vi "Memory.Pointer.Copy All.Unsafe.vi"(8 "error in (no error)":errorcluster, 10 "dst pointer in":refnum<class "Memory.Pointer.lvclass">, 11 "src pointer in":refnum<class "Memory.Pointer.lvclass">) -> (0 "error out":errorcluster, 2 "dst pointer out":refnum<class "Memory.Pointer.lvclass">, 3 "src pointer out":refnum<class "Memory.Pointer.lvclass">)   [LabVIEW 2016, in "Memory Manager.lvlib" / "Memory.Pointer.lvclass"]
doc: "Copies all of the data from the memory address pointed to by <b>src pointer</b> to the memory address pointed to by <b>dst pointer</b>.\n\n<b>Note:</b> This VI is <b>unsafe</b>.\n\nUnsafe means that this function does not have a check to ensure that the size of the source memory is inbounds of allocated memory for the destination before peforming a memory read/write. Reading/writing more data to a pointer than it has allocated can corrupt or crash LabVIEW. Only use this VI in scenarios where the <b>dst pointer</b> has been validated to be allocated to a correct size before calling this VI."
uses:
  Memory.Pointer.lvclass
  Memory.Pointer.lvclass/Memory.Pointer.ctl
  Memory.Pointer.Copy.Unsafe.vi
  Accessors/Get Address.vi
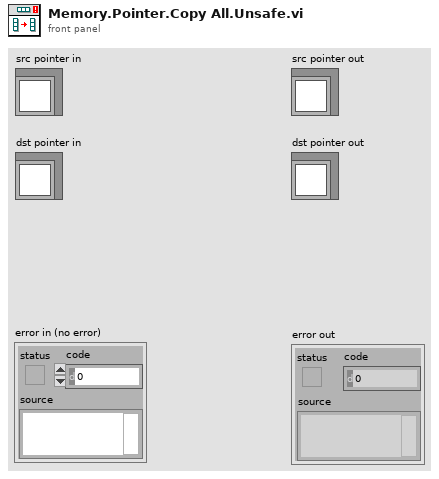
[diagram p1: front panel]
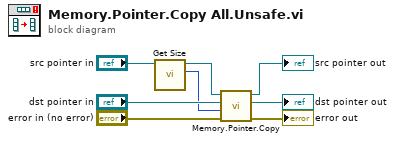
[diagram p0: block diagram]
diagram:
  n1 = call "Get Size.vi"("Pointer in"="src pointer in") -> ("size"=w1:u64, "Pointer out"=w5:refnum<class "Memory.Pointer.lvclass">)  [unwired: 8 in, 1 out]
  n2 = call-poly "Memory.Pointer.Copy.vi"("error in (no error)"="error in (no error)", "bytes to copy"=w1, "dst pointer in"="dst pointer in", "src pointer in"=w5) -> ("error out"=→"error out":errorcluster, "dst pointer out"=→"dst pointer out":refnum<class "Memory.Pointer.lvclass">, "src pointer out"=→"src pointer out":refnum<class "Memory.Pointer.lvclass">)  [unwired: 4 in, 1 out]
